vi "Initialise Globals.vi"(8 "error in (no error)":errorcluster) -> (0 "error out":errorcluster)   [LabVIEW 2019]
uses:
  Typedefs/Sensor Types.ctl
  Message Globals.vi
  UI/Controls/Pages Tab.ctl
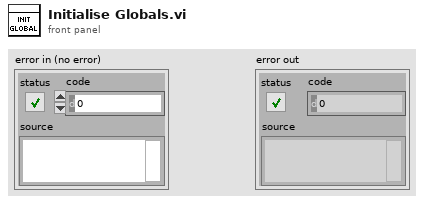
[diagram p1: front panel]
types:
  T1 = typedef "Pages Tab.ctl" = enum32{"Waiting", "Home"}
  T2 = typedef "Sensor Types.ctl" = enum16{"APP", "TURBIDITY", "PH"}
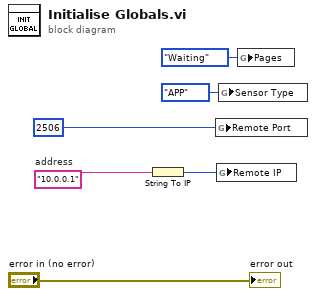
[diagram p0: block diagram]
diagram:
  w6 = "10.0.0.1"  # address
  n1 = String To IP(1:w6) -> (0:w4:u32)
  n2 = global write "Message Globals.vi" "Remote Port"(u16 2506 ("port or service name")) -> ()
  n3 = global write "Message Globals.vi" "Remote IP"(w4) -> ()
  n4 = global write "Message Globals.vi" "Sensor Type"(Sensor_Types."APP" ("Sensor Type")) -> ()
  n5 = global write "Message Globals.vi" "Pages"(Pages_Tab."Waiting" ("Pages")) -> ()
  "error out" <- "error in (no error)"
